vi "Class Adaptation Lesson 2.vi"() -> ()   [LabVIEW 2023]
doc: "Lesson 2 on the special adaptation that malleable VIs can do with LabVIEW classes. In this lesson, you will see that multiple interfaces defined by a malleable VI can be implemented by a single class."
uses:
  Compressor Cooler/Compressor Cooler.lvclass
  Thermal Test/Thermal Test.lvclass/Thermal Test.ctl
  46e75d11-427b-4f6b-998d-613f872e6eba.vi
  Thermal Test/Read Starting Temperature.vi
  Compressor Cooler/Cool Until Target.vi
  Thermal Test/Run Test.vi
  Compressor Cooler/Read Temperature.vi
  Thermal Test/Check Result.vi
panel:
  out "pass?":bool[](array[boolean])
  # "Overview: The previous lesson showed a malleable VI wired with its original classes and again wired with different, unrelated classes. In this lesson, you will see that multiple interfaces defined by a malleable VI can be implemented by a single class.\n\nInstructions: \n1. Open the block diagram of this VI. Review the lessons presented there.\n2. Run the VI to see the pass/fail results. Each time you run, the data is randomly generated. This means that, by design, as part of this demo, most iterations will see some failures.\n3. This ends this example. You may wish to explore this topic further by looking at another shipping example where this feature is used and compared against other LabVIEW programming techniques:\nexamples\\Channels\\Replacing The Function At The Heart Of An Algorithm At Run Time"
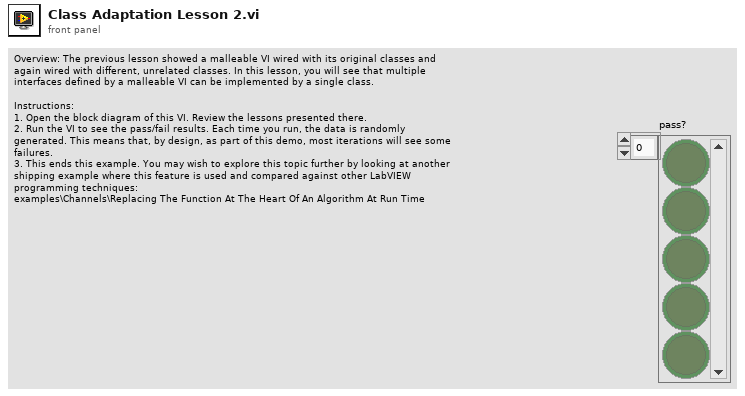
[diagram p1: front panel]
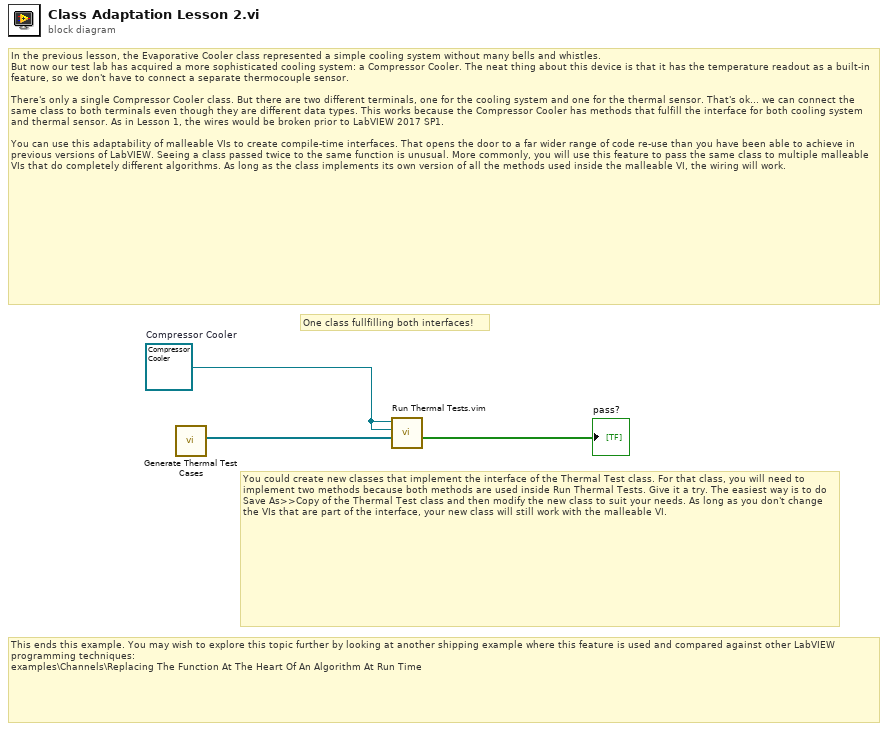
[diagram p0: block diagram]
diagram:
  w1 = refnum<class "Compressor Cooler.lvclass"> refnum  # Compressor Cooler
  # "This ends this example. You may wish to explore this topic further by looking at another shipping example where this feature is used and compared against other LabVIEW programming techniques:\nexamples\\Channels\\Replacing The Function At The Heart Of An Algorithm At Run Time"
  # "You could create new classes that implement the interface of the Thermal Test class. For that class, you will need to implement two methods because both methods are used inside Run Thermal Tests. Give it a try. The easiest way is to do Save As>>Copy of the Thermal Test class and then modify the new class to suit your needs. As long as you don't change the VIs that are part of the interface, your new class will still work with the malleable VI."
  # "One class fullfilling both interfaces!"
  # "In the previous lesson, the Evaporative Cooler class represented a simple cooling system without many bells and whistles. \nBut now our test lab has acquired a more sophisticated cooling system: a Compressor Cooler. The neat thing about this device is that it has the temperature readout as a built-in feature, so we don't have to connect a separate thermocouple sensor. \n\nThere's only a single Compressor Cooler class. But there are two different terminals, one for the cooling system and one for the thermal sensor. That's ok... we can connect the same class to both terminals even though they are different data types. This works because the Compressor Cooler has methods that fulfill the interface for both cooling system and thermal sensor. As in Lesson 1, the wires would be broken prior to LabVIEW 2017 SP1.\n\nYou can use this adaptability of malleable VIs to create compile-time interfaces. That opens the door to a far wider range of code re-use than you have been able to achieve in previous versions of LabVIEW. Seeing a class passed twice to the same function is unusual. More commonly, you will use this feature to pass the same class to multiple malleable VIs that do completely different algorithms. As long as the class implements its own version of all the methods used inside the malleable VI, the wiring will work."
  n1 = call "Generate Thermal Test Cases.vi"() -> ("Array"=w3:refnum<class "Thermal Test.lvclass">[])  [unwired: 11 in]
  n2 = call "Run Thermal Tests.vim"("array of tests"=w3, "thermal sensor"=w1, "cooling system"=w1) -> ("pass?"=→"pass?":bool[])  [unwired: 7 in, 1 out]
